vi "在表格前面插入行.vi"(8 "错误输入（无错误）":errorcluster, 10 "内容":string[](array[string]), 11 "引用输入":refnum<vi>) -> (0 "错误输出":errorcluster, 3 "引用输出":refnum<vi>)   [LabVIEW 2014, in "表格.lvlib"]
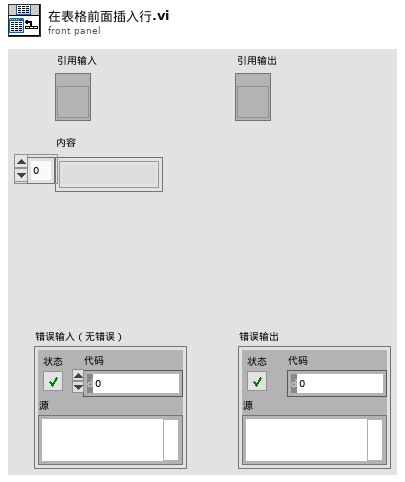
[diagram p1: front panel]
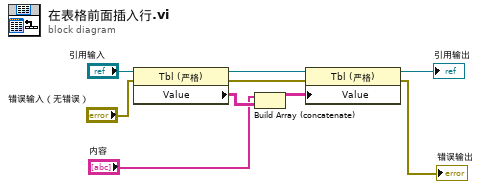
[diagram p0: block diagram]
diagram:
  n1 = property class="Tbl (严格)"(reference="引用输入", error in="错误输入（无错误）") -> (reference out=w8:refnum<vi>, error out=w7:errorcluster, "Value"=w2:string[][])
  n2 = Build Array (concatenate)("内容", w2) -> (w6:string[][])
  n3 = property class="Tbl (严格)"(reference=w8, error in=w7, "Value"=w6) -> (reference out=→"引用输出":refnum<vi>, error out=→"错误输出":errorcluster)
